vi "Set-parameter-lock.vi"(8 "error in (no error)":errorcluster, 9 "Lock?":bool, 11 "UI ref. in":refnum<data-value>) -> (0 "error out":errorcluster, 3 "UI ref.":refnum<data-value>)   [LabVIEW 2013, in "CameraVision.lvlib" / "CV-UI.lvclass"]
uses:
  CV-UI.lvclass
  CV-UI.lvclass/CV-UI.ctl
  Read Parameter refs.vi
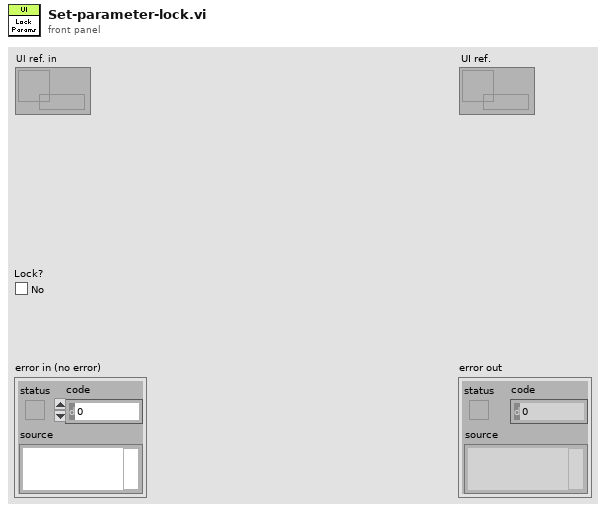
[diagram p1: front panel]
types:
  T1 = enum8{"Enabled", "Disabled", "Disabled and Grayed Out"}
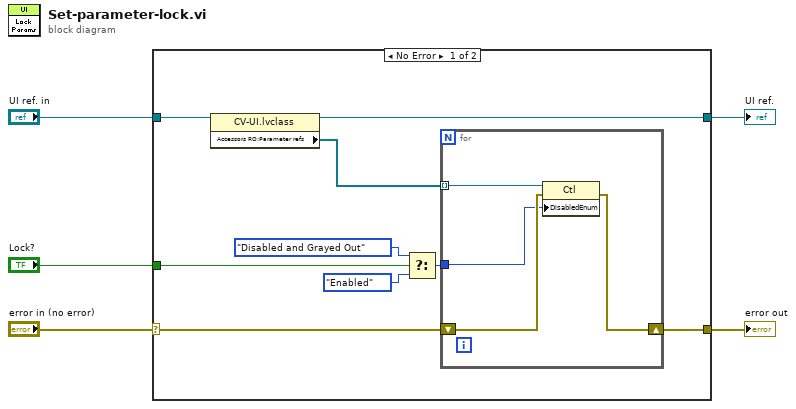
[diagram p0: block diagram]
diagram:
  n1 = case shown="No Error" "error in (no error)" {
    selector: "error in (no error)" -> [w11 w19]
    tunnel: [w13 w19] -> w4
    tunnel: [w12 w20] -> w2
    tunnel: "UI ref. in" -> [w14 w20]
    tunnel: "Lock?" -> [w10 _]
    frame No Error {
      n2 = property class="CV-UI.lvclass"(reference=w14) -> (reference out=w12:refnum<data-value>, "Accessors RO:Parameter refs"=w6:refnum<vi>[])  [unwired: 1 in, 1 out]
      n3 = Select(t=T1."Disabled and Grayed Out" ("Disabled"), s=w10, f=T1."Enabled" ("Disabled")) -> (s? t:f=w9:T1)
      n4 = for {
        tunnel: w9 -> [w16]
        shift-right: [w18] -> w13
        shift-left: w11 -> [w17]
        tunnel: w6 -> [w15] mode=indexing
        n5 = property class="Ctl"(reference=w15, error in=w17, "DisabledEnum"=w16) -> (error out=w18:errorcluster)  [unwired: 1 out]
      }
    }
    frame Error {
    }
  }
  "error out" <- w4
  "UI ref." <- w2
